vi "VisionTrig.vi"(8 "Constant I":dbl format="%#_13g", 9 "Omega":dbl format="%#_13g", 10 "Phi":dbl format="%#_13g", 11 "F constant":dbl format="%#_13g") -> (0 "Beta":dbl, 1 "Theta":dbl, 2 "Epsilon":dbl, 3 "Constant D":dbl)   [LabVIEW 2018]
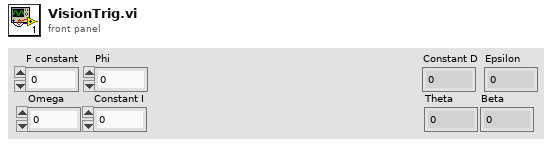
[diagram p1: front panel]
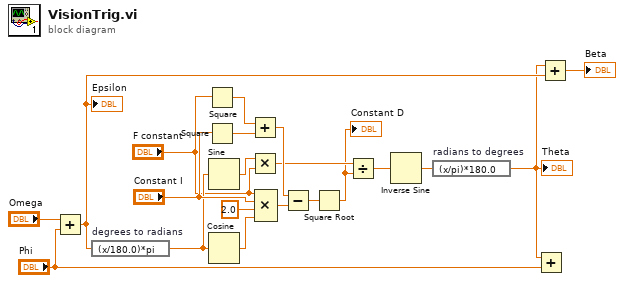
[diagram p0: block diagram]
diagram:
  n1 = Add(x="Omega", y="Phi") -> (x+y=w4:dbl)
  "Epsilon" <- w4
  n2 = expression code="(x/180.0)*pi" "degrees to radians"(w4) -> (w11:dbl)
  n3 = Square(x="F constant") -> (x^2=w19:dbl)
  n4 = Square(x="Constant I") -> (x^2=w18:dbl)
  n5 = Sine(x=w11) -> (sin(x)=w10:dbl)
  n6 = Cosine(x=w11) -> (cos(x)=w14:dbl)
  n7 = Add(x=w19, y=w18) -> (x+y=w17:dbl)
  n8 = Multiply(x=w10, y="F constant") -> (x*y=w8:dbl)
  n9 = Compound Arithmetic op=MULTIPLY("F constant", "Constant I", 2.0 ("value"), w14) -> (w13:dbl)
  n10 = Subtract(x=w17, y=w13) -> (x-y=w12:dbl)
  n11 = Square Root(x=w12) -> (sqrt(x)=w7:dbl)
  "Constant D" <- w7
  n12 = Divide(x=w8, y=w7) -> (x/y=w6:dbl)
  n13 = Inverse Sine(1:w6) -> (0:w5:dbl)
  n14 = expression code="(x/pi)*180.0" "radians to degrees"(w5) -> (w2:dbl)
  "Theta" <- w2
  n15 = Add(x=w2, y="Phi") -> ()  [unwired: 1 out]
  n16 = Add(x=w2, y=w4) -> (x+y=→"Beta":dbl)
